vi "Determine Confluence Connection.vi"(8 "Error in":errorcluster caption="Error in (no error)", 11 "Confluence Settings":T1) -> (0 "Error out":errorcluster, 3 "Confluence":refnum<class "Confluence.lvclass">)   [LabVIEW 2023]
uses:
  <userlib>/_PetranWay/LabVIEW Confluence API/Source/Confluence/Confluence Connection/Confluence.lvclass
  <userlib>/_PetranWay/LabVIEW Confluence API/Source/Data Center/Confluence Data Center/API/Construct Confluence Data Center.vi
  <userlib>/_PetranWay/LabVIEW Confluence API/Source/Data Center/Confluence Data Center/Confluence Data Center.lvclass
  <userlib>/_PetranWay/LabVIEW Confluence API/Source/Data Center/Confluence Data Center/API/Construct Confluence Data Center From Cache.vi
  <userlib>/_PetranWay/LabVIEW Confluence API/Source/Cloud/Confluence Cloud/API/Construct Confluence Cloud From Cache.vi
  <userlib>/_PetranWay/LabVIEW Confluence API/Source/Cloud/Confluence Cloud/Confluence Cloud.lvclass
  C:/Program Files/National Instruments/LabVIEW 2023/user.lib/_PetranWay/LabVIEW Confluence API/Source/Confluence/Confluence Connection/Confluence.lvclass
  C:/Program Files/National Instruments/LabVIEW 2023/user.lib/_PetranWay/LabVIEW Confluence API/Source/Confluence/iConfluence/iConfluence.lvclass
  C:/Program Files/National Instruments/LabVIEW 2023/user.lib/_PetranWay/LabVIEW Confluence API/Source/Data Center/Confluence Data Center/Confluence Data Center.lvclass
  C:/Program Files/National Instruments/LabVIEW 2023/user.lib/_PetranWay/LabVIEW Confluence API/Source/Cloud/Confluence Cloud/Confluence Cloud.lvclass
  <userlib>/_PetranWay/LabVIEW Confluence API/Source/Cloud/Confluence Cloud/API/Construct Confluence Cloud.vi
  Confluence Settings.ctl
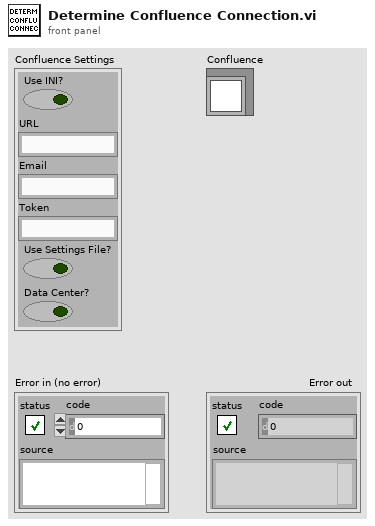
[diagram p1: front panel]
types:
  T1 = typedef "Confluence Settings.ctl" = cluster{"Use INI?":bool, "URL":string, "Email":string, "Token":string, "Use Settings File?":bool, "Data Center?":bool}
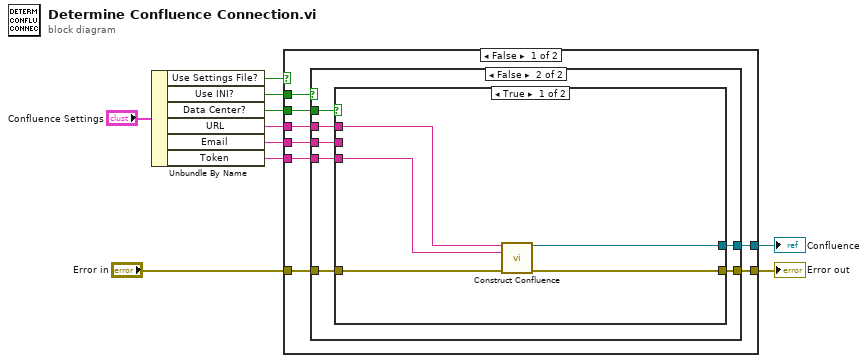
[diagram p0: block diagram]
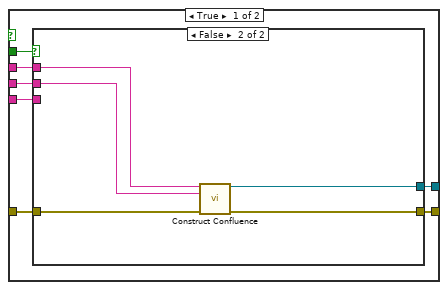
[diagram p2: hidden frame]
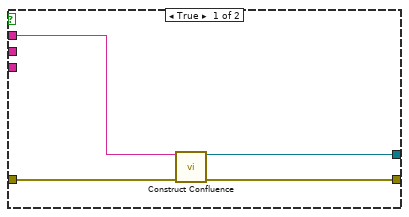
[diagram p3: hidden frame]
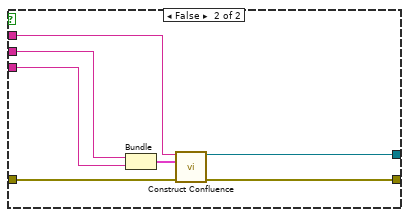
[diagram p4: hidden frame]
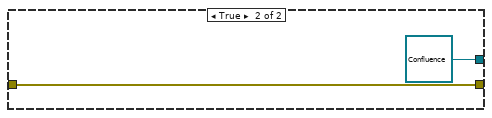
[diagram p5: hidden frame]
diagram:
  n1 = Unbundle By Name("Confluence Settings") -> ("Use Settings File?"=w9:bool, "Use INI?"=w6:bool, "Data Center?"=w5:bool, "URL"=w4:string, "Email"=w3:string, "Token"=w2:string)
  n2 = case shown="False" w9 {
    tunnel: [w12 w55] -> w8
    tunnel: "Error in" -> [w13 w55]
    tunnel: w6 -> [w18 _]
    tunnel: w5 -> [w17 _]
    tunnel: w4 -> [w16 _]
    tunnel: w3 -> [w15 _]
    tunnel: w2 -> [w14 _]
    tunnel: [w11 refnum<class "Confluence.lvclass"> refnum ("Confluence")] -> w1
    frame False {
      n3 = case shown="False" w18 {
        tunnel: w17 -> [w25 w41]
        tunnel: w16 -> [w24 w40]
        tunnel: w15 -> [w23 w39]
        tunnel: w14 -> [w22 w38]
        tunnel: w13 -> [w21 w37]
        tunnel: [w20 w36] -> w12
        tunnel: [w19 w35] -> w11
        frame True {
          n4 = case shown="False" w25 {
            tunnel: w24 -> [w26 w31]
            tunnel: w23 -> [_ w30]
            tunnel: w22 -> [_ _]
            tunnel: w21 -> [w29 w34]
            tunnel: [w28 w33] -> w20
            tunnel: [w27 w32] -> w19
            frame True {
              n5 = call-poly <userlib>:"Construct Confluence.vi"("Server URL"=w26, "error in (no error)"=w29) -> ("Confluence Data Center out"=w27:refnum<class "Confluence Data Center.lvclass">, "error out"=w28:errorcluster)  [unwired: 10 in, 2 out]
            }
            frame False {
              n6 = call-poly <userlib>:"Construct Confluence.vi"("Organization Name (https://[Organization Name].atlassian.net]"=w31, "Email Address"=w30, "error in (no error)"=w34) -> ("Confluence Cloud out"=w32:refnum<class "Confluence Cloud.lvclass">, "error out"=w33:errorcluster)  [unwired: 9 in, 2 out]
            }
          }
        }
        frame False {
          n7 = case shown="True" w41 {
            tunnel: w40 -> [w43 w50]
            tunnel: w39 -> [_ w49]
            tunnel: w38 -> [w42 w48]
            tunnel: w37 -> [w46 w53]
            tunnel: [w45 w52] -> w36
            tunnel: [w44 w51] -> w35
            frame True {
              n8 = call-poly <userlib>:"Construct Confluence.vi"("Your server URL"=w43, "Bearer Token"=w42, "error in (no error)"=w46) -> ("Confluence Data Center out"=w44:refnum<class "Confluence Data Center.lvclass">, "error out"=w45:errorcluster)  [unwired: 11 in]
            }
            frame False {
              n9 = Bundle("Email"=w49, "Token"=w48) -> (w47:cluster{"Email":string, "Token":string})  [unwired: 1 in]
              n10 = call-poly <userlib>:"Construct Confluence.vi"("Your Domain URL"=w50, "Email and Token"=w47, "error in (no error)"=w53) -> ("Confluence Cloud out"=w51:refnum<class "Confluence Cloud.lvclass">, "error out"=w52:errorcluster)  [unwired: 11 in]
            }
          }
        }
      }
    }
    frame True {
    }
  }
  "Error out" <- w8
  "Confluence" <- w1
